vi "RunTimeMenuUI.vi"() -> ()   [LabVIEW 2019, in "RunTimeMenuItem.lvclass"]
uses:
  RunTimeMenuItem.lvclass
  <vilib>/NI/Configuration Framework/Node/NodeRef.ctl
  <vilib>/NI/Configuration Framework/Node/NISE_CEF_Node.lvclass
  <vilib>/NI/AMC/Message Queue.ctl
  <vilib>/NI/AMC/Message.ctl
  <vilib>/NI/Tools/Keyed Array/KeyedArray.ctl
  <vilib>/NI/Configuration Framework/Node/UserEventRef.ctl
  <vilib>/NI/Configuration Framework/Controls/EventCluster.ctl
  C:/Program Files (x86)/National Instruments/LabVIEW 2019/vi.lib/NI/Configuration Framework/Node/NISE_CEF_Node.lvclass
  RunTimeMenuItem.lvclass/RunTimeMenuItem.ctl
  Read Run Time Menu Properties.vi
  Write Run Time Menu Properties.vi
  <vilib>/NI/AMC/Create Single Message.vi
  <vilib>/NI/AMC/Update Message Routing Info.vi
  <vilib>/NI/AMC/Send Message.vi
  <vilib>/NI/AMC/AMC.lvlib
  Configuration Tool.lvlib
  <vilib>/NI/Tools/Keyed Array/Tools_KeyedArray.lvlib
  <vilib>/NI/Configuration Framework/NISE_CEF_TreeControl.lvlib
panel:
  in  "Main UI Tab":T1(tab)
  in  "Name":string
  in  "GUID":string="9b525fa0-4d4a-4ec1-902b-bfeef88ebbcc"
  in  "Menu Item Type":enum16{"Action", "VI", "Separator", "Custom"}(ring)
  in  "Host Path to Menu VI":path
  in  "Host Path to Custom Menu Item":path
  in  "Execution":enum16{"silent", "modal", "floating", "default"}(ring)
  in  "Behavior":enum16{"Nothing", "Open Front Panel"}(ring)
  in  "Position":enum16{"Centered", "Mouse Pointer"}(ring)
  in  "Min # Of Children":u32
  in  "Host Path to Dependency File":path
  in  "Dependency Behavior":enum16{"Static", "Dynamic"}(ring)
  in  "user event":T2
  in  "main queue":T3
  in  "node ref":T4
  # "Display Settings"
  # "Dialog Settings"
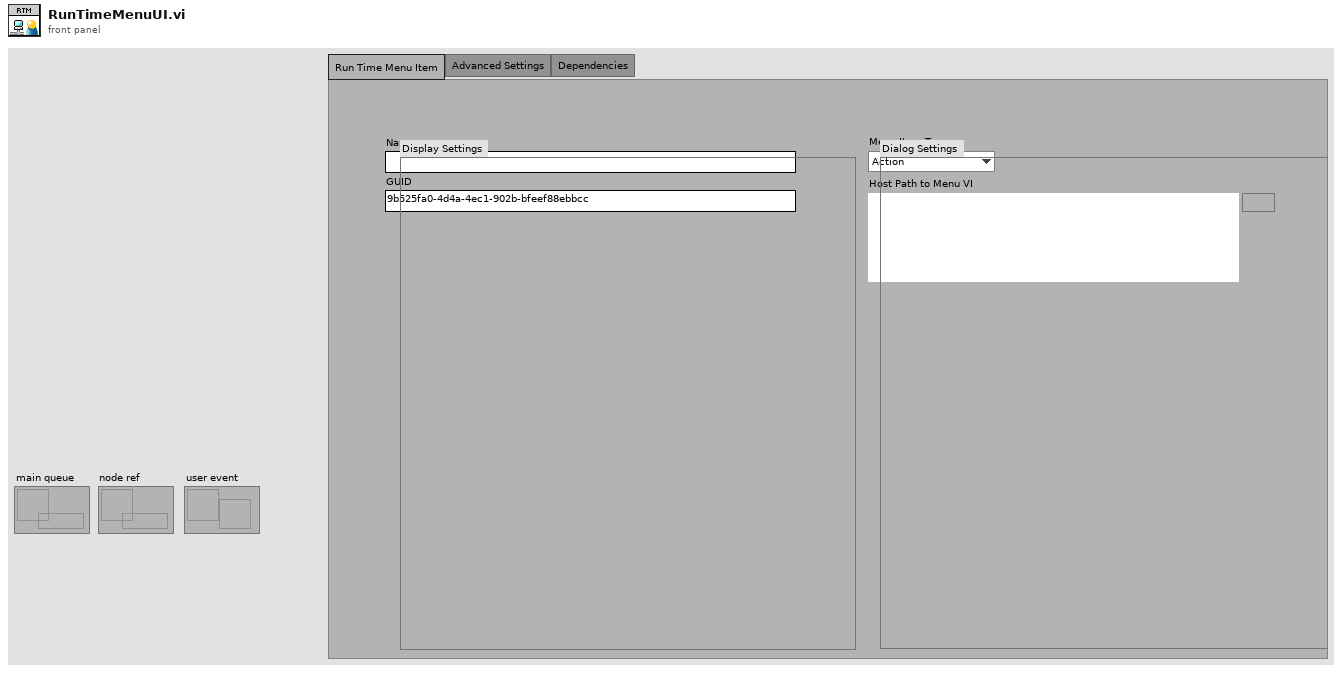
[diagram p1: front panel]
types:
  T1 = enum32{"Run Time Menu Item", "Advanced Settings", "Dependencies"}
  T2 = typedef "NISE_CEF_Node.lvclass/UserEventRef.ctl" = refnum<user-event>
  T3 = typedef "AMC.lvlib/Message Queue.ctl" = refnum<queue>
  T4 = typedef "NISE_CEF_Node.lvclass/NodeRef.ctl" = refnum<data-value>
  T5 = typedef "VeriStand Custom Device XML Parser.lvlib/RunTimeMenus Properties.ctl" = cluster{"GUID":string, "Execution":T6, "MinNrOfChilds":u32, "Name":string, "Item to Launch":T7, "Dependency":T8, "Custom Population":T7, "Menu Item Type":enum16{"Action", "VI", "Separator", "Custom"}, "Behavior":enum16{"Nothing", "Open Front Panel"}, "Position":enum16{"Centered", "Mouse Pointer"}}
  T6 = typedef "VeriStand Custom Device XML Parser.lvlib/Execution Types.ctl" = enum16{"silent", "modal", "floating", "default"}
  T7 = typedef "VeriStand Custom Device XML Parser.lvlib/Path Cluster.ctl" = cluster{"Path":path, "Path Type":enum16{"Absolute", "To Base", "To Common Doc Dir", "To Application Data Dir"}}
  T8 = typedef "VeriStand Custom Device XML Parser.lvlib/Dependency Properties.ctl" = cluster{"File Path Control":path, "Path Type":enum16{"Absolute", "To Base", "To Common Doc Dir", "To Application Data Dir"}, "Behavior":enum16{"Static", "Dynamic"}}
  T9 = enum16{"Absolute", "To Base", "To Common Doc Dir", "To Application Data Dir"}
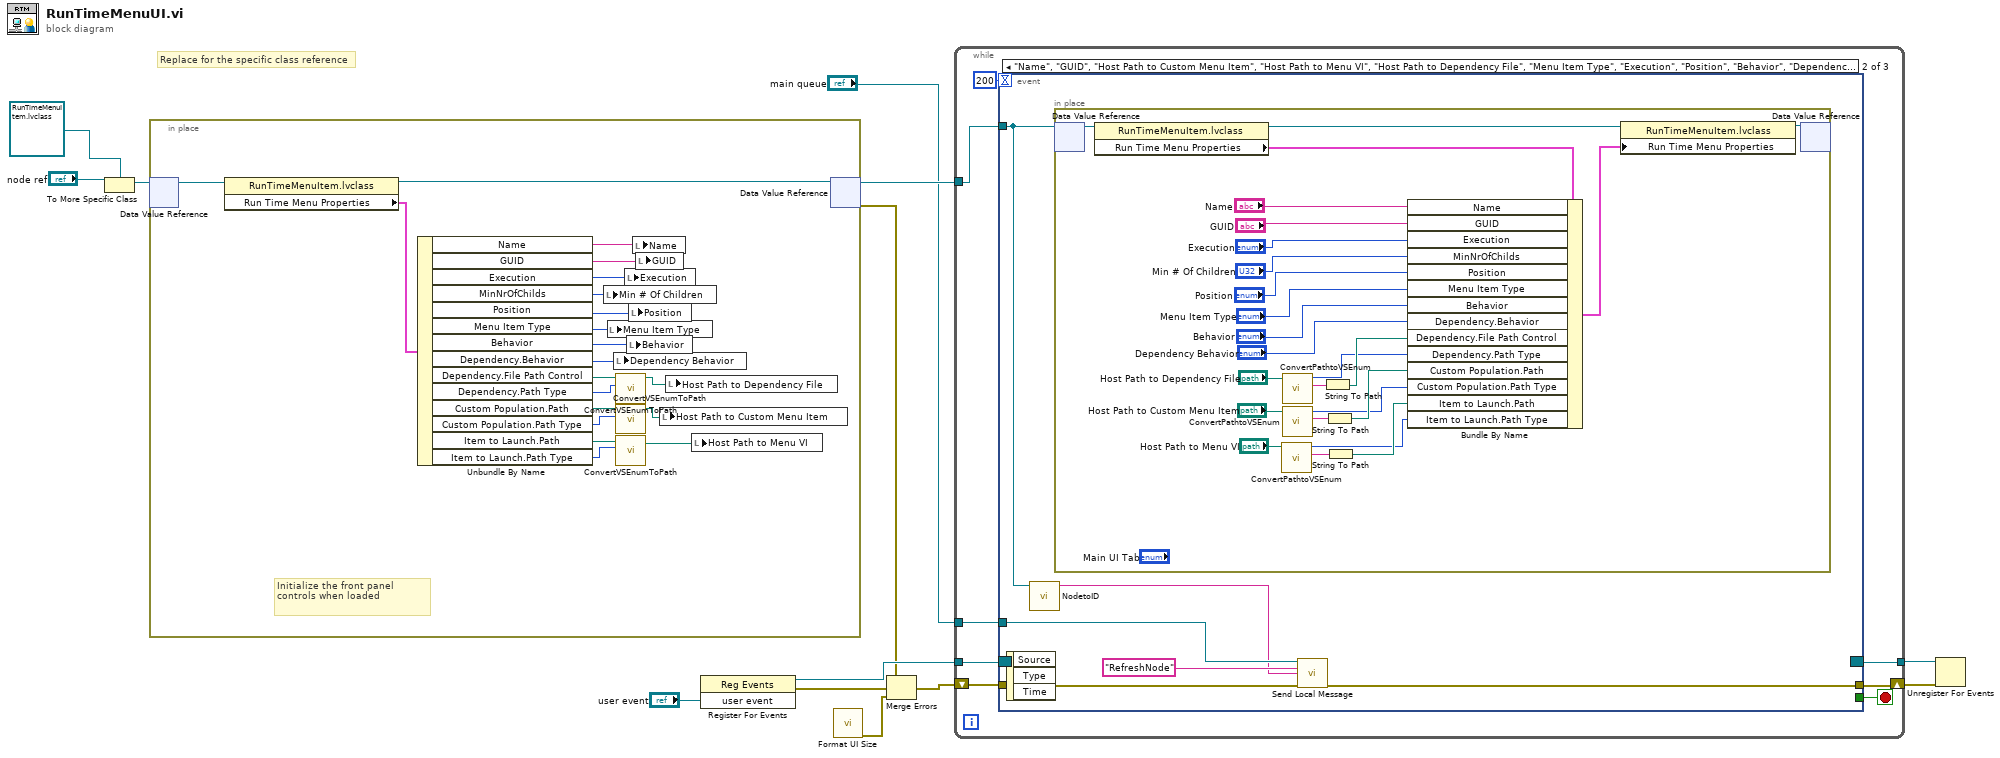
[diagram p0: block diagram]
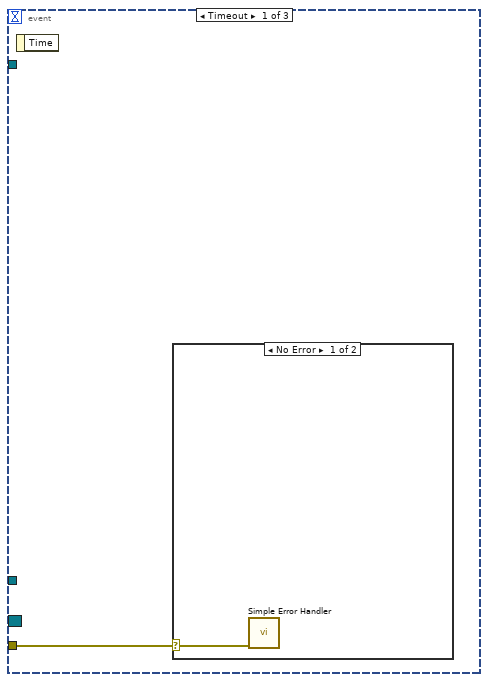
[diagram p2: hidden frame]
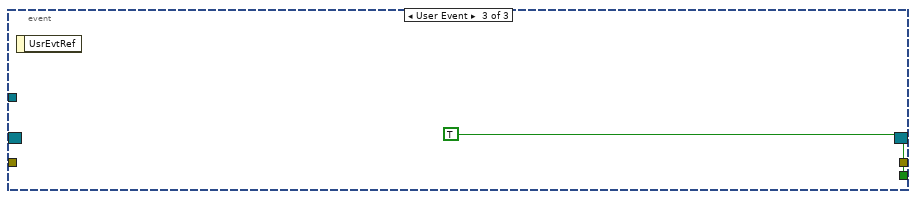
[diagram p4: hidden frame]
diagram:
  # "Replace for the specific class reference"
  n1 = To More Specific Class(target class=refnum<data-value> refnum ("data value reference"), reference="node ref") -> (specific class reference=w6:refnum<data-value>)  [unwired: 1 in, 1 out]
  n2 = in-place {
    # "Initialize the front panel controls when loaded"
    n3 = in-place-dvr #1(w6) -> (w33:refnum<class "RunTimeMenuItem.lvclass">)  [unwired: 1 out]
    n4 = property class="RunTimeMenuItem.lvclass"(reference=w33) -> (reference out=w32:refnum<class "RunTimeMenuItem.lvclass">, "Run Time Menu Properties"=w31:T5)  [unwired: 1 in, 1 out]
    n5 = Unbundle By Name(w31) -> ("Name"=w30:string, "GUID"=w29:string, "Execution"=w28:T6, "MinNrOfChilds"=w27:u32, "Position"=w26:enum16{"Centered", "Mouse Pointer"}, "Menu Item Type"=w25:enum16{"Action", "VI", "Separator", "Custom"}, "Behavior"=w24:enum16{"Nothing", "Open Front Panel"}, "Dependency.Behavior"=w23:enum16{"Static", "Dynamic"}, "Dependency.File Path Control"=w22:path, "Dependency.Path Type"=w21:T9, "Custom Population.Path"=w20:path, "Custom Population.Path Type"=w19:T9, "Item to Launch.Path"=w18:path, "Item to Launch.Path Type"=w17:T9)
    n6 = local write "Min # Of Children"(w27) -> ()
    n7 = local write "Menu Item Type"(w25) -> ()
    n8 = local write "Dependency Behavior"(w23) -> ()
    n9 = call "ConvertVSEnumToPath.vi"("Source.Path Type"=w21, "Path In"=w22) -> ("appended path"=w16:path)  [unwired: 9 in]
    n10 = call "ConvertVSEnumToPath.vi"("Source.Path Type"=w19, "Path In"=w20) -> ("appended path"=w15:path)  [unwired: 9 in]
    n11 = call "ConvertVSEnumToPath.vi"("Source.Path Type"=w17, "Path In"=w18) -> ("appended path"=w14:path)  [unwired: 9 in]
    n12 = local write "Execution"(w28) -> ()
    n13 = local write "Behavior"(w24) -> ()
    n14 = local write "Position"(w26) -> ()
    n15 = local write "Name"(w30) -> ()
    n16 = local write "GUID"(w29) -> ()
    n17 = local write "Host Path to Custom Menu Item"(w15) -> ()
    n18 = local write "Host Path to Dependency File"(w16) -> ()
    n19 = local write "Host Path to Menu VI"(w14) -> ()
    n20 = in-place-dvr #1(w32) -> (w13:refnum<data-value>, w3:errorcluster)
  }
  n21 = register-events("user event") -> (reference out=w10:refnum<event-registration>, error out=w4:errorcluster)  [unwired: 2 in]
  n22 = call "Format UI Size.vi"() -> ("error out"=w1:errorcluster)  [unwired: 11 in]
  n23 = Merge Errors(w3, w4, w1) -> (w2:errorcluster)
  n24 = while {
    tunnel: w13 -> [w41]
    tunnel: "main queue" -> [w40]
    tunnel: w10 -> [w38]
    tunnel: [w37] -> w9
    shift-right: [w35] -> w8
    shift-left: w2 -> [w34]
    stop <- w36 stop-if-true
    n25 = event shown="[1] \"Name\", \"GUID\", \"Host Path to Custom Menu Item\", \"Host Path to Menu VI\", \"Host Path to Dependency File\", \"Menu Item Type\", \"Execution\", \"Position\", \"Behavior\", \"Dependency Behavior\", \"Min # Of Children\": Value Change" {
      selector: w38 -> [_ _ _]
      dyn-events: [_ _ _] -> w37
      timeout: 200 -> [_ _ _]
      tunnel: w41 -> [_ w47 _]
      tunnel: w40 -> [_ w48 _]
      tunnel: [_ _ TRUE] -> w36
      tunnel: [_ w45 _] -> w35
      tunnel: w34 -> [w42 w44 _]
      event Timeout {
        n26 = event-data() -> ()  [unwired: 1 in, 1 out]
        n27 = case shown="No Error" w42 {
          selector: w42 -> [w43 _]
          frame No Error {
            n28 = call <vilib>:"Simple Error Handler.vi"("error in (no error)"=w43) -> ()  [unwired: 4 in, 5 out]
          }
          frame Error {
          }
        }
      }
      event "Name", "GUID", "Host Path to Custom Menu Item", "Host Path to Menu VI", "Host Path to Dependency File", "Menu Item Type", "Execution", "Position", "Behavior", "Dependency Behavior", "Min # Of Children": Value Change {
        n29 = event-data() -> ()  [unwired: 1 in, 3 out]
        n30 = call <vilib>:"NodetoID.vi"("node ref"=w47) -> ("ID"=w46:string)  [unwired: 9 in, 1 out]
        n31 = in-place {
          n32 = in-place-dvr #2(w47) -> (w72:refnum<class "RunTimeMenuItem.lvclass">)  [unwired: 1 out]
          n33 = property class="RunTimeMenuItem.lvclass"(reference=w72) -> (reference out=w71:refnum<class "RunTimeMenuItem.lvclass">, "Run Time Menu Properties"=w70:T5)  [unwired: 1 in, 1 out]
          n34 = call "ConvertPathtoVSEnum.vi"("Path In"="Host Path to Menu VI") -> ("Remaining Path"=w53:string, "VS Enum Out"=w51:T9)  [unwired: 9 in]
          n35 = call "ConvertPathtoVSEnum.vi"("Path In"="Host Path to Dependency File") -> ("Remaining Path"=w73:string, "VS Enum Out"=w59:T9)  [unwired: 9 in]
          n36 = call "ConvertPathtoVSEnum.vi"("Path In"="Host Path to Custom Menu Item") -> ("Remaining Path"=w57:string, "VS Enum Out"=w55:T9)  [unwired: 9 in]
          n37 = String To Path(string=w73) -> (path=w60:path)
          n38 = String To Path(string=w57) -> (path=w56:path)
          n39 = String To Path(string=w53) -> (path=w52:path)
          n40 = Bundle By Name(cluster=w70, "Name"="Name", "GUID"="GUID", "Execution"="Execution", "MinNrOfChilds"="Min # Of Children", "Position"="Position", "Menu Item Type"="Menu Item Type", "Behavior"="Behavior", "Dependency.Behavior"="Dependency Behavior", "Dependency.File Path Control"=w60, "Dependency.Path Type"=w59, "Custom Population.Path"=w56, "Custom Population.Path Type"=w55, "Item to Launch.Path"=w52, "Item to Launch.Path Type"=w51) -> (w50:T5)
          n41 = property class="RunTimeMenuItem.lvclass"(reference=w71, "Run Time Menu Properties"=w50) -> (reference out=w74:refnum<class "RunTimeMenuItem.lvclass">)  [unwired: 1 in, 1 out]
          n42 = in-place-dvr #2(w74) -> ()  [unwired: 2 out]
        }
        n43 = call <vilib>:"Send Local Message.vi"("message queue in"=w48, "message name"="RefreshNode" ("Message Name"), "message value"=w46, "error in"=w44) -> ("error out"=w45:errorcluster)  [unwired: 9 in, 2 out]
      }
      event User Event {
        n44 = event-data() -> ()  [unwired: 1 in, 1 out]
      }
    }
  }
  n45 = Unregister For Events(event registration refnum=w9, error in=w8) -> ()  [unwired: 1 out]
